vi "dfd_Get NStage Rational Resampling Filter Spec.vi"(5 "manual factorization in":T1[](array[typedef])=[{"L"=1, "M"=2}, {"L"=1, "M"=5}, {"L"=1, "M"=3}], 6 "fs in":dbl=3000.0, 7 "rational factor":T1={"L"=1, "M"=30}, 8 "error in":errorcluster, 9 "ripple specs":T2={"passband"=0.1, "stopband"=60.0, "dB/linear? (T: dB)"=TRUE}, 10 "freq specs [Hz]":T4={"fpass"=45.0, "fstop"=52.0}) -> (0 "error out":errorcluster, 1 "ripple specs (dB)":T2={"passband"=0.05437453093312722, "stopband"=0.001, "dB/linear? (T: dB)"=FALSE}, 2 "NStage freq specs [Hz]":T3[](array[typedef]), 3 "manual factorization out":T1[](array[typedef]), 4 "filter fs":dbl[](array[numeric]))   [LabVIEW 2017, in "NI_DigFilterLicensed.lvlib"]
uses:
  <vilib>/addons/Digital Filter Design/NI_DigFilterLicensed.lvlib
  <vilib>/addons/Digital Filter Design/_Objects.llb/DFD Multirate Rational Factor.ctl
  <vilib>/addons/Digital Filter Design/_Objects.llb/DFD Filter Ripple Specification (Design).ctl
  <vilib>/addons/Digital Filter Design/_Objects.llb/DFD Multirate Filter Specification (Design).ctl
  <vilib>/addons/Digital Filter Design/_Objects.llb/DFD Filter Frequence Specification (Design).ctl
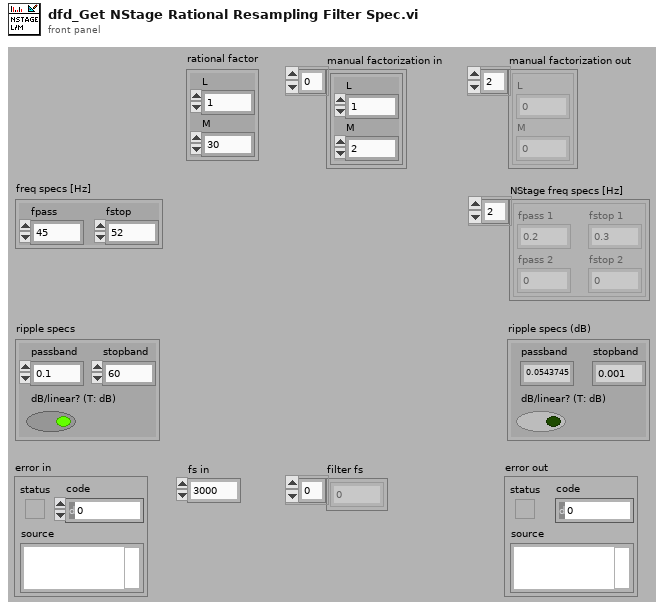
[diagram p1: front panel]
types:
  T1 = typedef "NI_DigFilterLicensed.lvlib/DFD Multirate Rational Factor.ctl" = cluster{"L":i32, "M":i32}
  T2 = typedef "NI_DigFilterLicensed.lvlib/DFD Filter Ripple Specification (Design).ctl" = cluster{"passband":dbl, "stopband":dbl, "dB/linear? (T: dB)":bool}
  T3 = typedef "NI_DigFilterLicensed.lvlib/DFD Filter Frequence Specification (Design).ctl" = cluster{"fpass 1":dbl, "fstop 1":dbl, "fpass 2 ":dbl, "fstop 2":dbl}
  T4 = typedef "NI_DigFilterLicensed.lvlib/DFD Multirate Filter Specification (Design).ctl" = cluster{"fpass":dbl, "fstop":dbl}
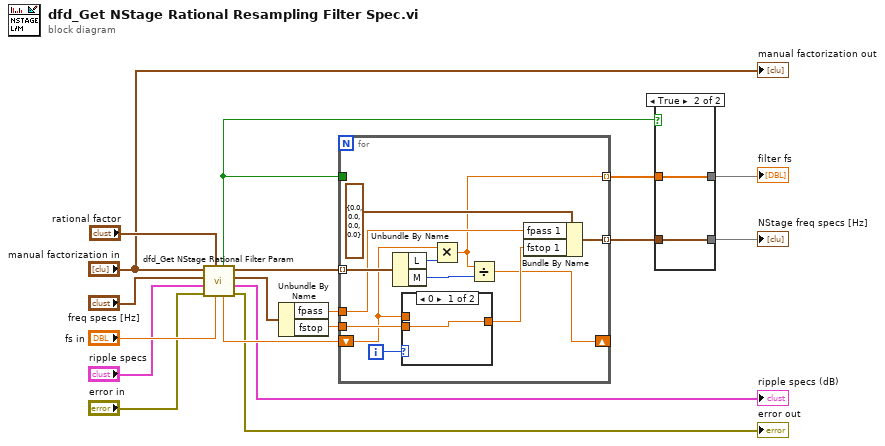
[diagram p0: block diagram]
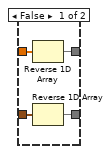
[diagram p2: hidden frame]
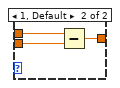
[diagram p3: hidden frame]
diagram:
  n1 = call <vilib>:"dfd_Get NStage Rational Filter Param.vi"("fs in"="fs in", "factor"="rational factor", "error in (no error)"="error in", "ripple specs"="ripple specs", "freq specs"="freq specs [Hz]", "manual factorization in"="manual factorization in") -> ("error out"=→"error out":errorcluster, "ripple specs (dB)"=→"ripple specs (dB)":T2, "dup freq specs"=w7:T4, "manual factorization out"=w15:T1[], "fs in"=w16:dbl, "interpolation/decimation?"=w4:bool)
  n2 = Unbundle By Name(w7) -> ("fpass"=w10:dbl, "fstop"=w11:dbl)
  n3 = for {
    shift-right: [w24] -> _
    shift-left: w16 -> [w22]
    tunnel: w10 -> [w26]
    tunnel: w11 -> [w29]
    tunnel: w15 -> [w28] mode=indexing
    tunnel: w4 -> [_]
    tunnel: [w21] -> w3 mode=indexing
    tunnel: [w19] -> w1 mode=indexing
    i -> [w30]
    n4 = Unbundle By Name(w28) -> ("L"=w23:i32, "M"=w27:i32)
    n5 = case shown="0" w30 {
      tunnel: w29 -> [w31 w34]
      tunnel: [w31 w33] -> w25
      tunnel: w22 -> [_ w32]
      frame 0 {
      }
      frame 1, Default {
        n6 = Subtract(x=w32, y=w34) -> (x-y=w33:dbl)
      }
    }
    n7 = Multiply(x=w22, y=w23) -> (x*y=w19:dbl)
    n8 = Divide(x=w19, y=w27) -> (x/y=w24:dbl)
    n9 = Bundle By Name(cluster=T3 {"fpass 1"=0.0, "fstop 1"=0.0, "fpass 2 "=0.0, "fstop 2"=0.0} ("freq specs [Hz] 2"), "fpass 1"=w26, "fstop 1"=w25) -> (w21:T3)
  }
  n10 = case shown="True" w4 {
    tunnel: [w38 w39] -> w5
    tunnel: w3 -> [w37 w40]
    tunnel: [w36 w40] -> w2
    tunnel: w1 -> [w35 w39]
    frame False {
      n11 = Reverse 1D Array(array=w35) -> (reversed array=w38:dbl[])
      n12 = Reverse 1D Array(array=w37) -> (reversed array=w36:T3[])
    }
    frame True {
    }
  }
  "NStage freq specs [Hz]" <- w2
  "filter fs" <- w5
  "manual factorization out" <- "manual factorization in"
